vi "Actividad_3.vi"() -> ()   [LabVIEW 2020]
panel:
  out "Waveform Chart":dynamicdata(graph)
  in  "Cantidad de muestras":dbl(slide) scale=0.0..500.0
  in  "Tiempo para realizar muestras (s)":dbl(slide) scale=0.0..10.0
  out "Voltaje":dbl
  in  "stop":bool
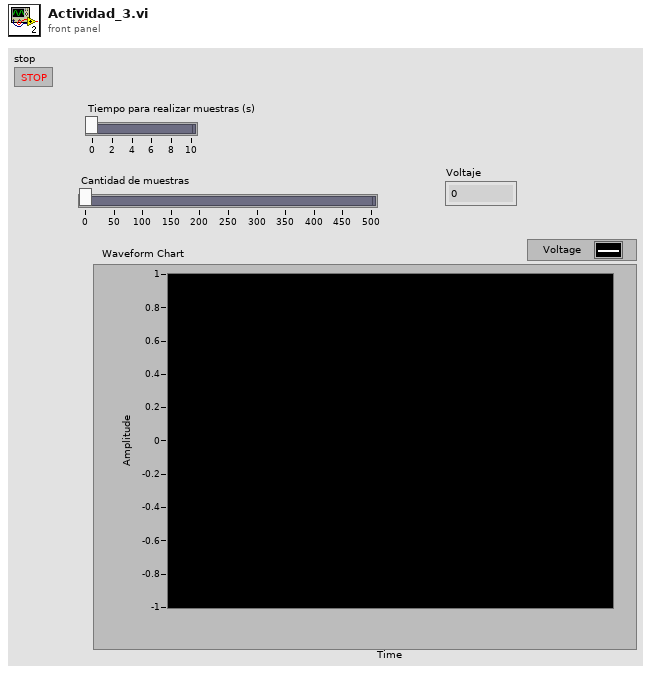
[diagram p1: front panel]
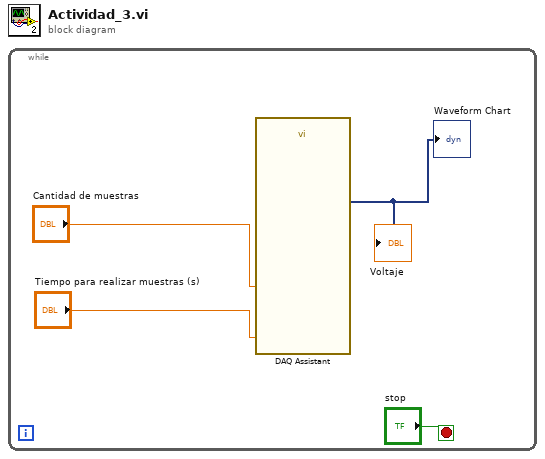
[diagram p0: block diagram]
diagram:
  n1 = while {
    stop <- "stop" stop-if-true
    n2 = call "DAQ Assistant"("number of samples"="Cantidad de muestras", "timeout (s)"="Tiempo para realizar muestras (s)") -> ("data"=→"Voltaje" →"Waveform Chart":dynamicdata)  [unwired: 15 in, 2 out]
  }
